vi "Get DiffArgFilepath.vi"(8 "error in (no error)":errorcluster) -> (0 "error out":errorcluster, 2 "VICompare Difftool Exe Path":path)   [LabVIEW 2016]
doc: "Find the location of the VICompare difftool EXE to be able to later parse the Diff Argument Booleans.\nIf Sourcetree is not used or VI Compare is not configured then output no path.\n\nLooks into the .getconfig file - first finding the .getconfig gile. If does not exist, path = empty.\n[difftool \"sourcetree\"] is inserted by Sourcetree into the gitconfig (expected). if this is not found path = empty.\n[ ] lines can be treated as config file sections - the key cmd will list the launch command to launch the External Diff tool.\nexpected to be cmd = 'C:/viscc/vidiff.exe' \\\"LOCAL\\\" \\\"$REMOTE\\\"\n\nThis VI should return C:\\viscc as the path, correcting the / to \\ for Windows.\n\nIf the above section or key are not found, path = empty."
uses:
  <vilib>/Utility/sysdir.llb/System Directory Type.ctl
  <vilib>/Utility/config.llb/Read Key (String).vi
  <vilib>/regexp/Match Regular Expression.xnode
  <vilib>/Utility/config.llb/NI_LVConfig.lvlib
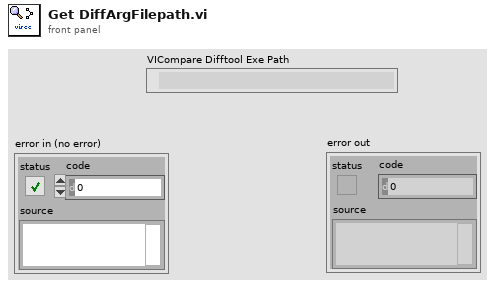
[diagram p1: front panel]
types:
  T1 = typedef "System Directory Type.ctl" = i32
  T2 = typedef "NI_LVConfig.lvlib/Config Data RefNum.ctl" = refnum<k1>
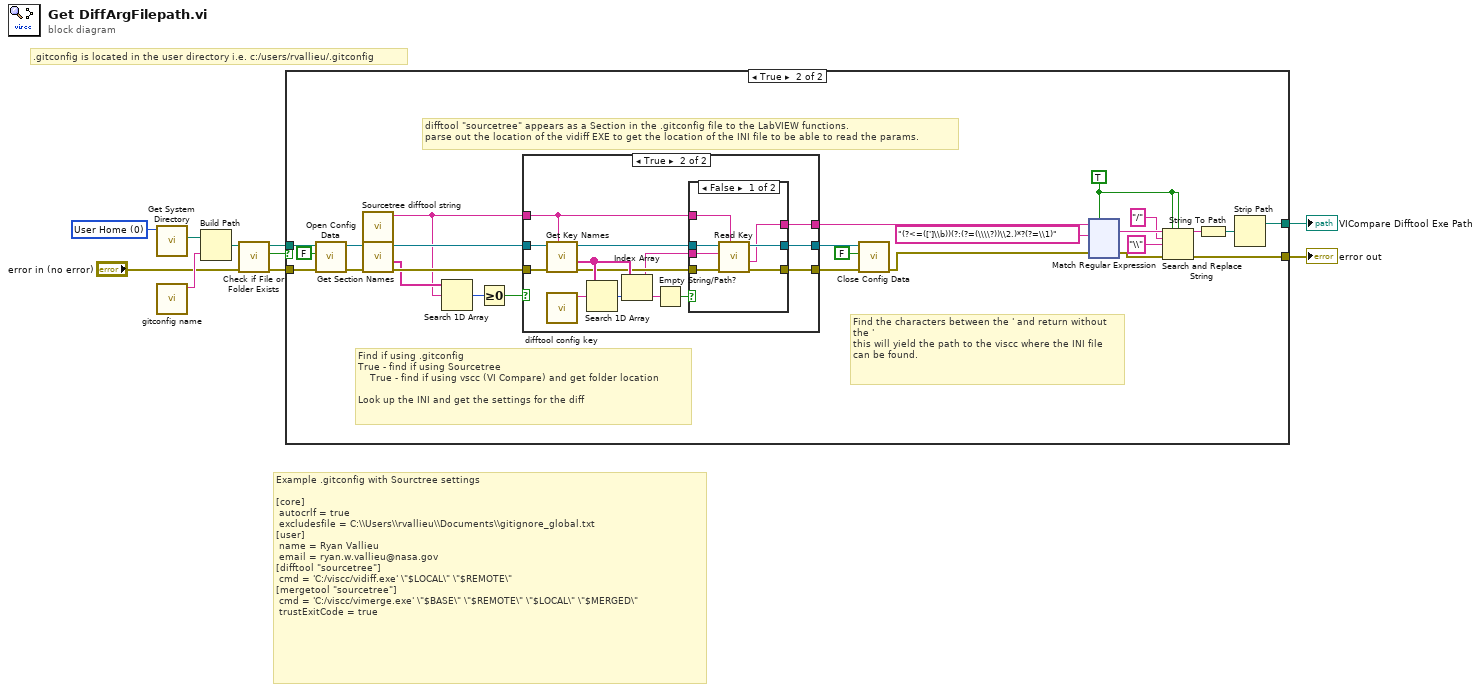
[diagram p0: block diagram]
diagram:
  w10 = T1 0 items=["User Home"=0, "User Desktop"=1, "User Documents"=2, "User Application Data"=3, "User Preferences"=4, "User Temporary"=5, "Public Documents"=6, "Public Application Data"=7, "Public Preferences"=8, "Public Cache"=13, "System Core Libraries"=9, "System Installed Libraries"=10, "Application Files"=11, "Boot Volume Root"=12] ("system directory type")
  # "Example .gitconfig with Sourctree settings\n\n[core]\n\tautocrlf = true\n\texcludesfile = C:\\\\Users\\\\rvallieu\\\\Documents\\\\gitignore_global.txt\n[user]\n\tname = Ryan Vallieu\n\temail = ryan.w.vallieu@nasa.gov\n[difftool \"sourcetree\"]\n\tcmd = 'C:/viscc/vidiff.exe' \\\"$LOCAL\\\" \\\"$REMOTE\\\"\n[mergetool \"sourcetree\"]\n\tcmd = 'C:/viscc/vimerge.exe' \\\"$BASE\\\" \\\"$REMOTE\\\" \\\"$LOCAL\\\" \\\"$MERGED\\\"\n\ttrustExitCode = true"
  # ".gitconfig is located in the user directory i.e. c:/users/rvallieu/.gitconfig"
  n1 = call <vilib>:"Get System Directory.vi"("system directory type"=w10) -> ("system directory"=w9:path)  [unwired: 10 in]
  n2 = call "gitconfig name.vi"() -> ("gitconfig filename"=w8:string)  [unwired: 11 in]
  n3 = Build Path(base path=w9, name or relative path=w8) -> (appended path=w7:path)
  n4 = call <vilib>:"Check if File or Folder Exists.vi"("error in (no error)"="error in (no error)", "path"=w7) -> ("error out"=w5:errorcluster, "file or folder exists?"=w2:bool, "dup path"=w6:path)  [unwired: 7 in]
  n5 = case shown="True" w2 {
    tunnel: w6 -> [_ w37]
    tunnel: w5 -> [w11 w25]
    tunnel: [w11 w18] -> w4
    tunnel: [_ w13] -> w3
    frame False {
    }
    frame True {
      w16 = TRUE ("ignore case? (F)")
      # "Find the characters between the ' and return without the '\nthis will yield the path to the viscc where the INI file can be found."
      # "difftool \"sourcetree\" appears as a Section in the .gitconfig file to the LabVIEW functions.\nparse out the location of the vidiff EXE to get the location of the INI file to be able to read the params."
      # "Find if using .gitconfig\nTrue - find if using Sourcetree\n    True - find if using vscc (VI Compare) and get folder location\n\nLook up the INI and get the settings for the diff"
      n6 = call <vilib>:"Open Config Data.vi"("error in (no error)"=w25, "create file if necessary (T)"=FALSE, "configuration file path"=w37) -> ("error out"=w30:errorcluster, "refnum"=w36:T2)  [unwired: 6 in, 1 out]
      n7 = call "Sourcetree difftool string.vi"() -> ("Sourcetree Difftool String"=w12:string)  [unwired: 11 in]
      n8 = call <vilib>:"Get Section Names.vi"("error in (no error)"=w30, "refnum"=w36) -> ("error out"=w31:errorcluster, "section names"=w28:string[], "refnum out"=w33:T2)  [unwired: 7 in]
      n9 = Search 1D Array(1D array=w28, element=w12) -> (index of element=w27:i32)  [unwired: 1 in]
      n10 = Greater Or Equal To 0?(x=w27) -> (x >= 0?=w26:bool)
      n11 = case shown="True" w26 {
        tunnel: w33 -> [w153 w166]
        tunnel: [w153 w161] -> w32
        tunnel: w31 -> [w152 w164]
        tunnel: [w152 w159] -> w29
        tunnel: w12 -> [_ w155]
        tunnel: [_ w156] -> w23
        frame False {
        }
        frame True {
          n12 = call <vilib>:"Get Key Names.vi"("section"=w155, "error in (no error)"=w164, "refnum"=w166) -> ("error out"=w160:errorcluster, "key names"=w162:string[], "refnum out"=w165:T2)  [unwired: 5 in, 1 out]
          n13 = call "difftool config key.vi"() -> ("difftool key"=w154:string)  [unwired: 11 in]
          n14 = Search 1D Array(1D array=w162, element=w154) -> (index of element=w163:i32)  [unwired: 1 in]
          n15 = Index Array(array=w162, index=w163) -> (element=w158:string)
          n16 = Empty String/Path?(string/path=w158) -> (empty?=w157:bool)
          n17 = case shown="False" w157 {
            tunnel: w165 -> [w173 w175]
            tunnel: [w172 w175] -> w161
            tunnel: w160 -> [w171 w174]
            tunnel: [w170 w174] -> w159
            tunnel: w158 -> [w169 _]
            tunnel: [w168 _] -> w156
            tunnel: w155 -> [w167 _]
            frame False {
              n18 = call-poly <vilib>:"Read Key.vi"("section"=w167, "error in (no error)"=w171, "key"=w169, "refnum"=w173) -> ("error out"=w170:errorcluster, "value"=w168:string, "refnum out"=w172:T2)  [unwired: 4 in, 1 out]
            }
            frame True {
            }
          }
        }
      }
      n19 = call <vilib>:"Close Config Data.vi"("error in (no error)"=w29, "write file if changed (T)"=FALSE, "refnum"=w32) -> ("error out"=w19:errorcluster)  [unwired: 7 in, 1 out]
      n20 = xnode "Match Regular Expression"("input string"=w23, "regular expression"="(?<=([']\\b))(?:(?=(\\\\?))\\2.)*?(?=\\1)", "error in"=w19, "ignore case? (F)"=w16) -> ("whole match"=w22:string, "error out"=w17:errorcluster)  [unwired: 2 in, 3 out]
      n21 = Search and Replace String(replace all?=w16, case sensitive?=w16, input string=w22, search string="/", replace string="\\" ("replace string (\"\")"), error in=w17) -> (result string=w20:string, error out=w18:errorcluster)  [unwired: 2 in, 2 out]
      n22 = String To Path(string=w20) -> (path=w14:path)
      n23 = Strip Path(path=w14) -> (stripped path=w13:path)  [unwired: 1 out]
    }
  }
  "error out" <- w4
  "VICompare Difftool Exe Path" <- w3
